vi "Read_Motor_modified.vi"(8 "error in (no error)":errorcluster, 10 "Motor ID (0)":u8, 11 "VISA Refnum in":refnum<visa-resource-name>) -> (0 "error out":errorcluster, 2 "Position":dbl, 3 "VISA Refnum out":refnum<visa-resource-name>)   [LabVIEW 2015]
uses:
  <instrlib>/Dynamixel Motor/Dynamixel Motor.lvlib
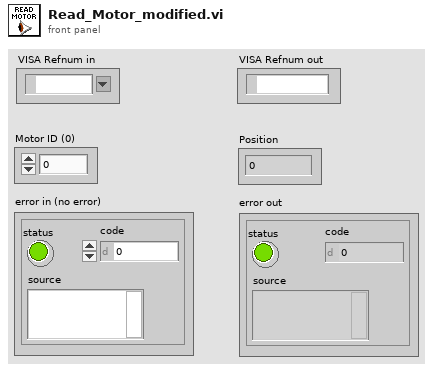
[diagram p1: front panel]
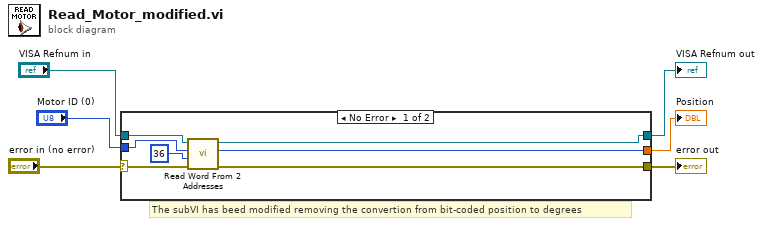
[diagram p0: block diagram]
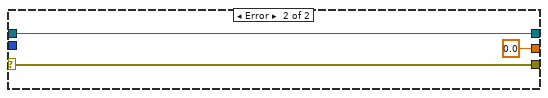
[diagram p2: hidden frame]
diagram:
  # "The subVI has beed modified removing the convertion from bit-coded position to degrees"
  n1 = case shown="No Error" "error in (no error)" {
    selector: "error in (no error)" -> [w8 w15]
    tunnel: "VISA Refnum in" -> [w13 w16]
    tunnel: [w12 w16] -> w1
    tunnel: [w11 w15] -> w6
    tunnel: [w7 0.0] -> w5
    tunnel: "Motor ID (0)" -> [w10 _]
    frame No Error {
      n2 = call <instrlib>:"Read Word From 2 Addresses.vi"("Error in (no error)"=w8, "Address number (0)"=u8 36 ("Address # DEC"), "Motor ID (0)"=w10, "VISA resource name"=w13) -> ("error out"=w11:errorcluster, "Data"=w7:u16, "VISA resource name out"=w12:refnum<visa-resource-name>)  [unwired: 5 in]
    }
    frame Error {
    }
  }
  "error out" <- w6
  "Position" <- w5
  "VISA Refnum out" <- w1
